vi "Printing Process.vi"(8 "error in (no error)":errorcluster, 11 "Domino Laser module Class in":refnum<class "Domino Laser module Class.lvclass">) -> (0 "error out":errorcluster, 3 "Domino Laser module Class out":refnum<class "Domino Laser module Class.lvclass">)   [LabVIEW 2015, in "Domino LM.lvlib" / "Domino Laser module Class.lvclass"]
uses:
  CTRLS/Domino Laser module Class.lvclass
  ORG_SRL_CTRL/Queue Enum.ctl
  CTRLS/GLB_VAR.vi
  ORG_SRL_CTRL/WO Operation Enum.ctl
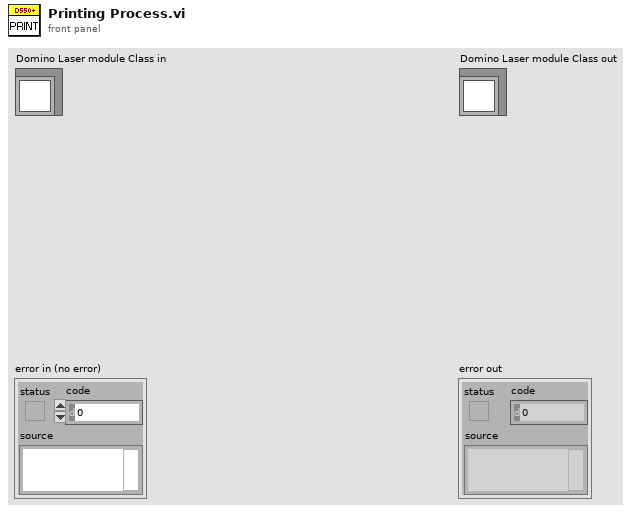
[diagram p1: front panel]
types:
  T1 = enum16{"Send variable to print", "Wait for print end", "INIT"}
  T2 = typedef "WO Operation Enum.ctl" = enum16{"Get Batch Data", "Update Batch Data", "Start Batch", "Stop Batch", "Check Batch"}
  T3 = typedef "Queue Enum.ctl" = enum16{"DB", "Notify", "Acquire", "Process", "PLC", "Printer", "Printer B", "Scanner A", "XML_DL", "EXC"}
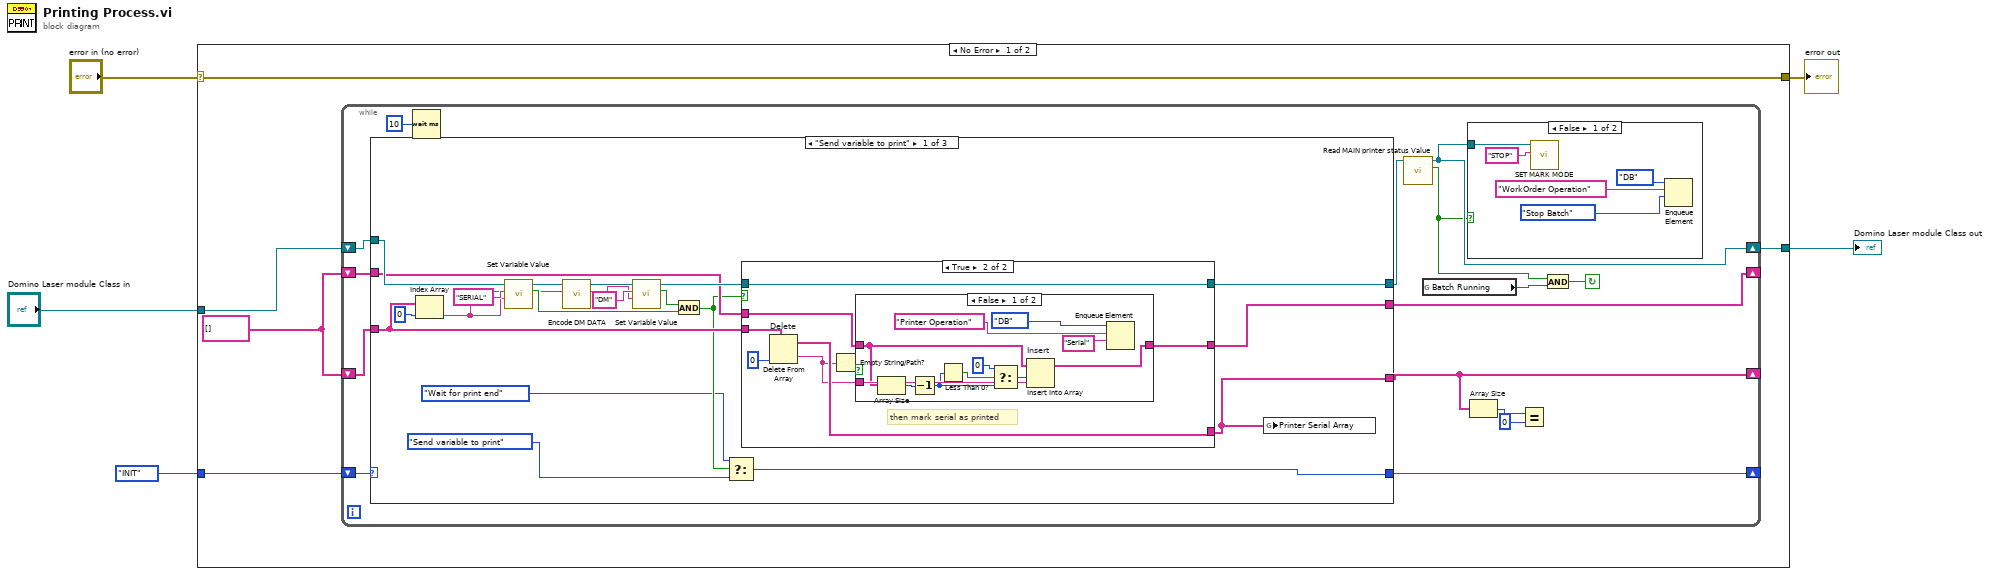
[diagram p0: block diagram]
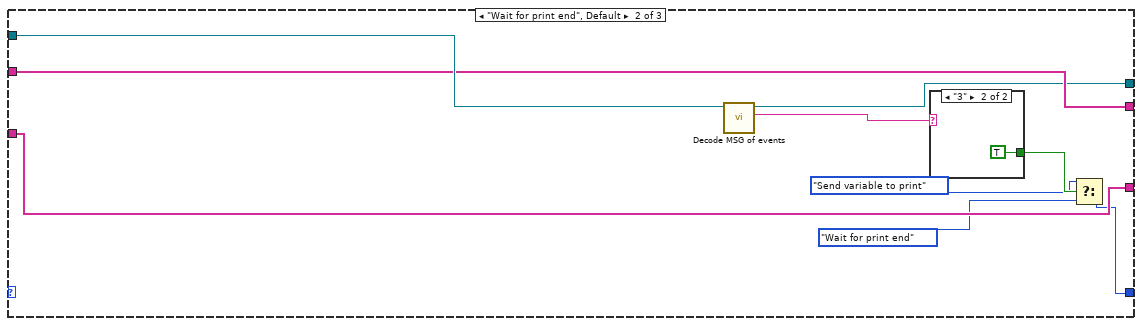
[diagram p5: hidden frame]
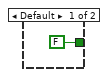
[diagram p6: hidden frame]
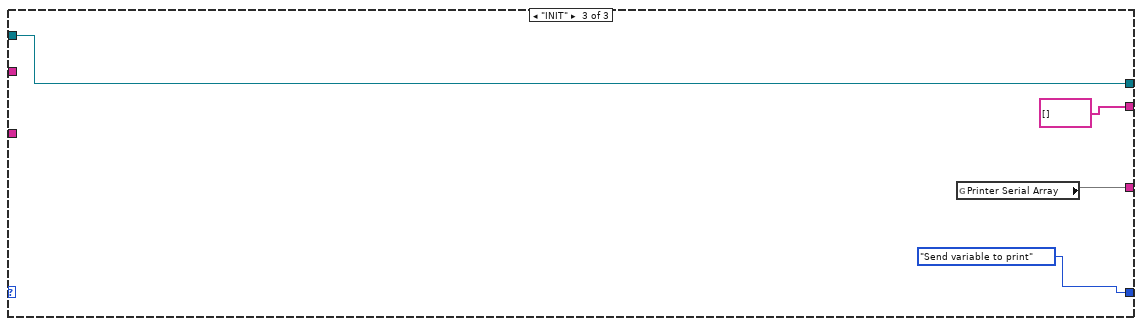
[diagram p7: hidden frame]
diagram:
  n1 = case shown="No Error" "error in (no error)" {
    selector: "error in (no error)" -> [w10 w90]
    tunnel: [w10 w90] -> w4
    tunnel: [w8 w89] -> w2
    tunnel: "Domino Laser module Class in" -> [w9 w89]
    tunnel: T1."INIT" ("Enum") -> [w7 _]
    frame No Error {
      w6 = string[] [] ("Seials array")
      n2 = while {
        shift-right: [w20] -> w8
        shift-left: w9 -> [w25]
        shift-right: [w13] -> _
        shift-left: w6 -> [w24]
        shift-right: [w22] -> _
        shift-left: w6 -> [w23]
        shift-right: [w18] -> _
        shift-left: w7 -> [w19]
        stop <- w14 continue-if-true
        n3 = case shown="\"Send variable to print\"" w19 {
          tunnel: w25 -> [w50 w82 w87]
          tunnel: [w46 w77 w87] -> w21
          tunnel: w24 -> [w44 w79 _]
          tunnel: w23 -> [w43 w78 _]
          tunnel: [w31 w78 string[] [] ("Seials array")] -> w22
          tunnel: [w36 w79 w86] -> w13
          tunnel: [w37 w74 T1."Send variable to print" ("Enum")] -> w18
          frame "Send variable to print" {
            n4 = Index Array(array=w44, index=0) -> (element=w35:string)
            n5 = call "Set Variable Value.vi"("VAR Value"=w35, "VAR NAME"="SERIAL", "Domino Laser module Class in"=w50) -> ("Var changed successfully?"=w41:bool, "Domino Laser module Class out"=w34:refnum<class "Domino Laser module Class.lvclass">)  [unwired: 6 in, 1 out]
            n6 = call "Encode DM DATA.vi"("serial"=w35, "Domino Laser module Class in"=w34) -> ("DM"=w32:string, "Domino Laser module Class out"=w33:refnum<class "Domino Laser module Class.lvclass">)  [unwired: 7 in, 1 out]
            n7 = call "Set Variable Value.vi"("VAR Value"=w32, "VAR NAME"="DM", "Domino Laser module Class in"=w33) -> ("Var changed successfully?"=w42:bool, "Domino Laser module Class out"=w45:refnum<class "Domino Laser module Class.lvclass">)  [unwired: 6 in, 1 out]
            n8 = And(x=w42, y=w41) -> (x .and. y?=w40:bool)
            n9 = Select(t=T1."Wait for print end" ("Enum"), s=w40, f=T1."Send variable to print" ("Enum")) -> (s? t:f=w37:T1)
            n10 = case shown="True" w40 {
              tunnel: [w53 w61] -> w46
              tunnel: w45 -> [w53 w61]
              tunnel: w44 -> [w52 w58]
              tunnel: w43 -> [w51 w59]
              tunnel: [w52 w57] -> w36
              tunnel: [w51 w56] -> w31
              frame False {
              }
              frame True {
                # "then mark serial as printed"
                n11 = Delete From Array "Delete"(array=w58, index=0) -> (deleted portion=w55:string, array with subset deleted=w57:string[])  [unwired: 1 in]
                n12 = Empty String/Path?(string/path=w55) -> (empty?=w54:bool)
                n13 = case shown="False" w54 {
                  tunnel: w55 -> [w72 _]
                  tunnel: w59 -> [w67 w73]
                  tunnel: [w71 w73] -> w56
                  frame False {
                    n14 = Array Size(array=w67) -> (size(s)=w66:i32)
                    n15 = Decrement(x=w66) -> (x-1=w64:i32)
                    n16 = Less Than 0?(x=w64) -> (x < 0?=w65:bool)
                    n17 = Select(t=0, s=w65, f=w64) -> (s? t:f=w62:i32)
                    n18 = Insert Into Array "Insert"(array=w67, index=w62, new element=w72) -> (w71:string[])
                    n19 = Enqueue Element(queue=Queue_Enum."DB" ("Enum"), element="Printer Operation" ("Message"), timeout in ms (-1)="Serial" ("Message")) -> ()  [unwired: 1 in, 3 out]
                  }
                  frame True {
                  }
                }
              }
            }
            n20 = global write "GLB_VAR.vi" "Printer Serial Array"(w36) -> ()
          }
          frame "Wait for print end", Default {
            n21 = call "Decode MSG of events.vi"("Domino Laser module Class in"=w82) -> ("MSG ID"=w81:string, "Domino Laser module Class out"=w77:refnum<class "Domino Laser module Class.lvclass">)  [unwired: 7 in, 2 out]
            n22 = case shown="\"3\"" w81 {
              tunnel: [FALSE TRUE] -> w80
              frame Default {
              }
              frame "3" {
              }
            }
            n23 = Select(t=T1."Send variable to print" ("Enum"), s=w80, f=T1."Wait for print end" ("Enum")) -> (s? t:f=w74:T1)
          }
          frame "INIT" {
            n24 = global read "GLB_VAR.vi" "Printer Serial Array"() -> (w86)
          }
        }
        n25 = Wait (ms)(milliseconds to wait=u32 10) -> ()  [unwired: 1 out]
        n26 = call "Read MAIN printer status Value.vi"("Domino Laser module Class in"=w21) -> ("Print stat"=w15:bool, "Domino Laser module Class out"=w20:refnum<class "Domino Laser module Class.lvclass">)  [unwired: 8 in, 1 out]
        n27 = global read "GLB_VAR.vi" "Batch Running"() -> (w16:bool)
        n28 = case shown="False" w15 {
          tunnel: w20 -> [w28 _]
          frame False {
            n29 = call "SET MARK MODE.vi"("mark mode"="STOP", "Domino Laser module Class in"=w28) -> ()  [unwired: 8 in, 2 out]
            n30 = Enqueue Element(queue=Queue_Enum."DB" ("Enum"), element="WorkOrder Operation" ("Message"), timeout in ms (-1)=WO_Operation_Enum."Stop Batch") -> ()  [unwired: 1 in, 3 out]
          }
          frame True {
          }
        }
        n31 = Array Size(array=w13) -> (size(s)=w12:i32)
        n32 = Equal?(x=w12, y=0) -> ()  [unwired: 1 out]
        n33 = And(x=w15, y=w16) -> (x .and. y?=w14:bool)
      }
    }
    frame Error {
    }
  }
  "error out" <- w4
  "Domino Laser module Class out" <- w2
